vi "Init.vi"(6 "parametrs ref":refnum<vi>, 7 "IP Adress in":string="192.168.0.200", 8 "Stop Event":refnum<user-event>, 9 "control_Pair ref":refnum<vi>, 10 "control_Port_2 ref":refnum<vi>, 11 "control_Port_1 ref":refnum<vi>) -> (0 "error out":errorcluster, 3 "Управление ПЛК":T1)   [LabVIEW 2023, in "pump_Lib.lvlib"]
uses:
  pump_Lib.lvlib
  TypeDef/control_Type.ctl
  TypeDef/pump_Type.ctl
  TypeDef/pair_Type.ctl
  TypeDef/parametrs_Type.ctl
panel:
  # "%"
  # "%"
  # "%"
  # "%"
  # "%"
  # "%"
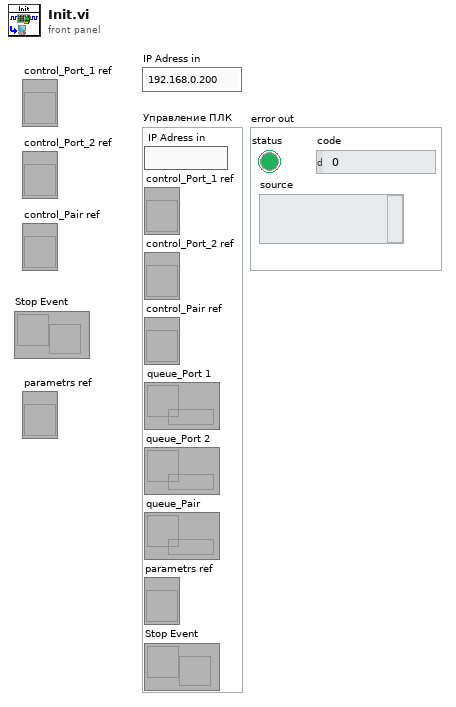
[diagram p1: front panel]
types:
  T1 = typedef "pump_Lib.lvlib/control_Type.ctl" = cluster{"IP Adress in":string, "control_Port_1 ref":refnum<vi>, "control_Port_2 ref":refnum<vi>, "control_Pair ref":refnum<vi>, "queue_Port 1":refnum<queue>, "queue_Port 2":refnum<queue>, "queue_Pair":refnum<queue>, "parametrs ref":refnum<vi>, "Stop Event":refnum<user-event>}
  T2 = typedef "pump_Lib.lvlib/pump_Type.ctl" = cluster{"Давление заданное":dbl, "Давление MAX заданное":dbl, "Давление в насосе":dbl, "Давление в системе":dbl, "Расход заданый":dbl, "Расход текущий":dbl, "Объём заданный":dbl, "Объём текущий":dbl, "Позиция насоса %":dbl, "Ток двигателя":dbl, "controlMsg":string, "Клапан k_sys":bool, "Клапан k_res":bool, "Клапан k_air":bool, "Вверх":bool, "Домой":bool, "Вниз":bool, "Старт расход":bool, "Старт давление":bool, "Сброс объёма":bool, "Сброс давления Рсис":bool, "Сброс давления Рнас":bool, "Bits":cluster{"plc_control":bool, "lag_control":bool, "mstop_control":bool, "st_home":bool, "error":bool, "mstart":bool, "pair":bool, "startQ":bool, "startP":bool, "volume_Stop":bool}}
  T3 = typedef "pump_Lib.lvlib/pair_Type.ctl" = cluster{"Давление заданное":dbl, "Давление в системе":dbl, "Расход заданый":dbl, "Расход текущий":dbl, "Объём заданный":dbl, "Объём текущий":dbl, "Старт давление":bool, "Старт расход":bool, "Сброс объёма":bool, "plc_control":bool, "lag_control":bool, "mstop_control":bool, "Давление":cluster{"АЦП CH 0":dbl, "АЦП CH 1":dbl, "АЦП CH 2":dbl, "АЦП CH 3":dbl, "АЦП CH 4":dbl, "АЦП CH 5":dbl, "АЦП CH 6":dbl, "АЦП CH 7":dbl}, "Modbus":cluster{"Массив чтения":u16[], "Массив записи":u16[]}}
  T4 = enum16{"open", "replace", "create", "open or create", "replace or create", "replace or create with confirmation"}
  T5 = enum16{"big-endian, network order", "native, host order", "little-endian"}
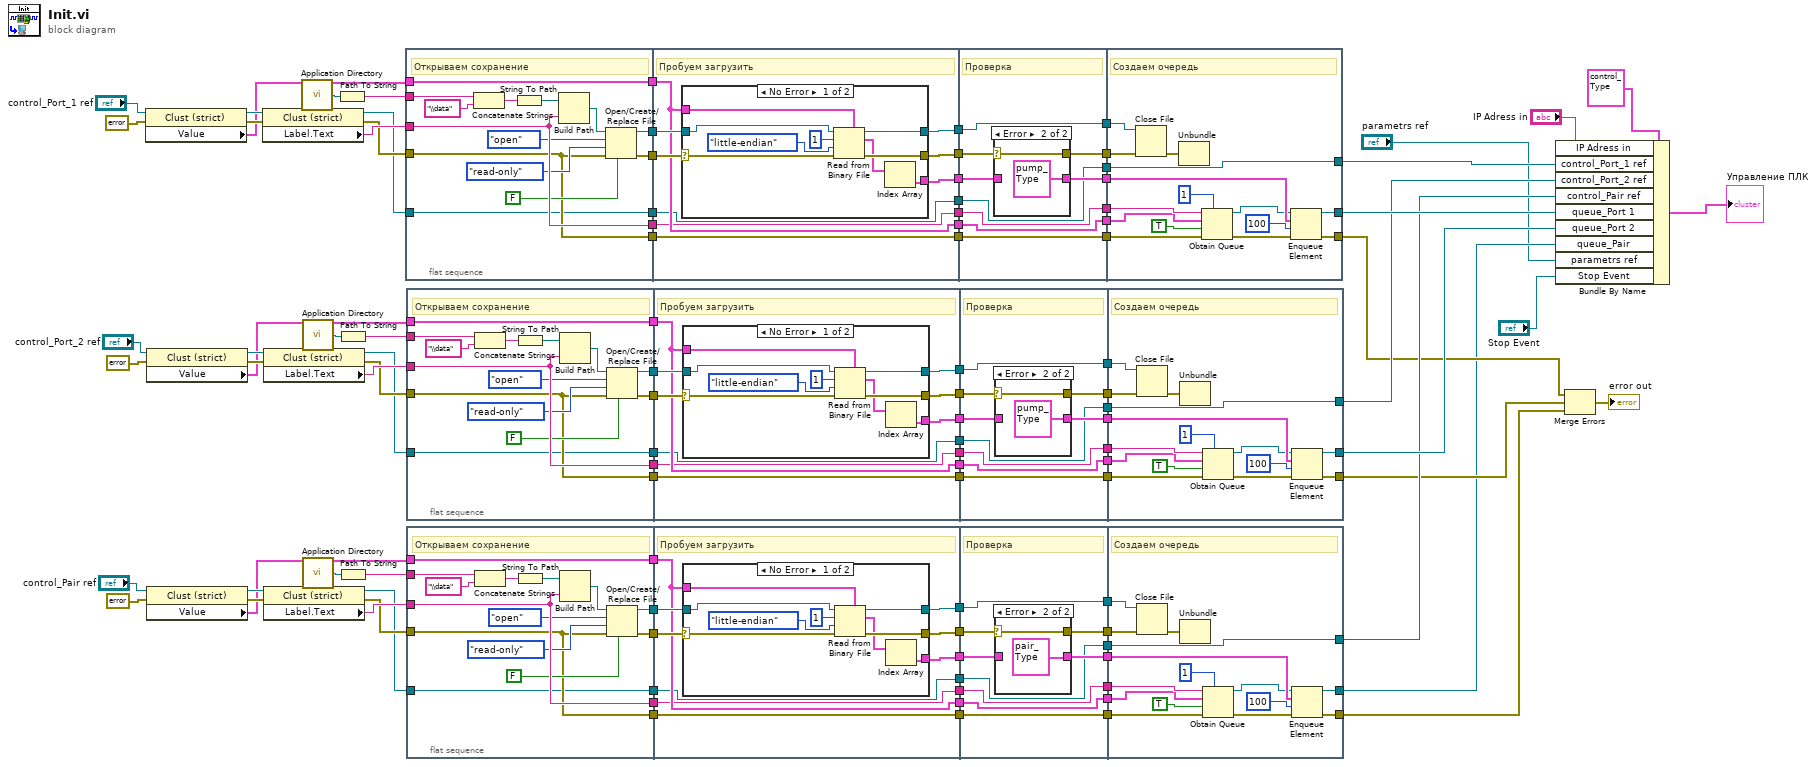
[diagram p0: block diagram]
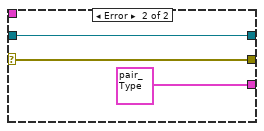
[diagram p2: hidden frame]
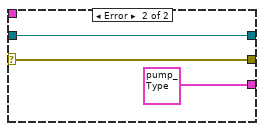
[diagram p4: hidden frame]
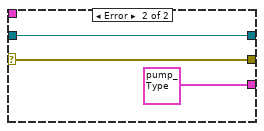
[diagram p6: hidden frame]
diagram:
  n1 = property class="Clust (strict)"(reference="control_Port_1 ref", error in=errorcluster {"status"=FALSE, "code"=0, "source"=""} ("error in (no error)")) -> (reference out=w99:refnum<vi>, error out=w100:errorcluster, "Value"=w77:T2)
  n2 = property class="Clust (strict)"(reference="control_Port_2 ref", error in=errorcluster {"status"=FALSE, "code"=0, "source"=""} ("error in (no error)")) -> (reference out=w47:refnum<vi>, error out=w48:errorcluster, "Value"=w45:T2)
  n3 = property class="Clust (strict)"(reference="control_Pair ref", error in=errorcluster {"status"=FALSE, "code"=0, "source"=""} ("error in (no error)")) -> (reference out=w18:refnum<vi>, error out=w19:errorcluster, "Value"=w16:T3)
  n4 = property class="Clust (strict)"(reference=w99, error in=w100) -> (reference out=w73:refnum<vi>, error out=w74:errorcluster, "Label.Text"=w76:string)
  n5 = property class="Clust (strict)"(reference=w47, error in=w48) -> (reference out=w42:refnum<vi>, error out=w43:errorcluster, "Label.Text"=w44:string)
  n6 = property class="Clust (strict)"(reference=w18, error in=w19) -> (reference out=w13:refnum<vi>, error out=w14:errorcluster, "Label.Text"=w15:string)
  n7 = call <vilib>:"Application Directory.vi"() -> ("Application Directory"=w102:path)
  n8 = call <vilib>:"Application Directory.vi"() -> ("Application Directory"=w50:path)
  n9 = call <vilib>:"Application Directory.vi"() -> ("Application Directory"=w21:path)
  n10 = Path To String(path=w102) -> (string=w78:string)
  n11 = Path To String(path=w50) -> (string=w46:string)
  n12 = Path To String(path=w21) -> (string=w17:string)
  n13 = flat-sequence {
    tunnel: w76 -> [w115]
    tunnel: [w115] -> w98
    tunnel: [w119] -> w97
    tunnel: w77 -> [w119]
    tunnel: w74 -> [w108]
    tunnel: w78 -> [w118]
    tunnel: [w110] -> w96
    tunnel: [w109] -> w95
    tunnel: [w108] -> w94
    tunnel: w73 -> [w106]
    tunnel: [w106] -> w93
    tunnel: w98 -> [w125]
    tunnel: w97 -> [w126]
    tunnel: w96 -> [w128]
    tunnel: w95 -> [w127]
    tunnel: [w126] -> w92
    tunnel: [w125] -> w91
    tunnel: [w124] -> w90
    tunnel: [w123] -> w89
    tunnel: [w122] -> w88
    tunnel: w94 -> [w122]
    tunnel: [w121] -> w87
    tunnel: w93 -> [w121]
    tunnel: [w120] -> w86
    tunnel: w92 -> [w149]
    tunnel: w91 -> [w148]
    tunnel: w90 -> [w146]
    tunnel: w89 -> [w147]
    tunnel: [w149] -> w85
    tunnel: [w148] -> w84
    tunnel: [w145] -> w83
    tunnel: w88 -> [w145]
    tunnel: [w144] -> w82
    tunnel: [w143] -> w81
    tunnel: w87 -> [w143]
    tunnel: [w142] -> w80
    tunnel: [w141] -> w79
    tunnel: w86 -> [w141]
    tunnel: w85 -> [w166]
    tunnel: w84 -> [w167]
    tunnel: w83 -> [w164]
    tunnel: w82 -> [w163]
    tunnel: w81 -> [w158]
    tunnel: [w160] -> w6
    tunnel: [w159] -> w72
    tunnel: [w158] -> w71
    tunnel: w80 -> [w157]
    tunnel: w79 -> [w156]
    frame #0 {
      # "Открываем сохранение"
      n14 = Concatenate Strings(w118, "\\data" ("string")) -> (w117:string)
      n15 = String To Path(string=w117) -> (path=w107:path)
      n16 = Build Path(base path=w107, name or relative path=w115) -> (appended path=w114:path)
      n17 = Open/Create/Replace File(file path (use dialog)=w114, error in=w108, operation (0:open)=T4."open", access (0:read/write)=enum16{"read/write", "read-only", "write-only"}."read-only", disable buffering (F)=FALSE) -> (refnum out=w109:refnum<file>, error out=w110:errorcluster)  [unwired: 1 in, 1 out]
    }
    frame #1 {
      # "Пробуем загрузить"
      n18 = case shown="No Error" w128 {
        selector: w128 -> [w136 w140]
        tunnel: w127 -> [w137 w139]
        tunnel: w126 -> [w135 _]
        tunnel: [w130 T2 {"Давление заданное"=0.3, "Давление MAX заданное"=100.0, "Давление в насосе"=0.0, "Давление в системе"=99.99, "Расход заданый"=0.0, "Расход текущий"=0.0, "Объём заданный"=0.0, "Объём текущий"=0.0, "Позиция насоса %"=0.0, "Ток двигателя"=0.0, "controlMsg"="", "Клапан k_sys"=FALSE, "Клапан k_res"=FALSE, "Клапан k_air"=FALSE, "Вверх"=FALSE, "Домой"=FALSE, "Вниз"=FALSE, "Старт расход"=FALSE, "Старт давление"=FALSE, "Сброс объёма"=FALSE, "Сброс давления Рсис"=FALSE, "Сброс давления Рнас"=FALSE, "Bits"={"plc_control"=FALSE, "lag_control"=FALSE, "mstop_control"=FALSE, "st_home"=FALSE, "error"=FALSE, "mstart"=FALSE, "pair"=FALSE, "startQ"=FALSE, "startP"=FALSE, "volume_Stop"=FALSE}} ("Насос")] -> w124
        tunnel: [w132 w140] -> w123
        tunnel: [w129 w139] -> w120
        frame No Error {
          n19 = Read from Binary File(5:w135, 8:w136, 9:T5."little-endian" ("byte order (0:big-endian, network order)"), 10:1 ("count (1)"), 11:w137) -> (0:w132:errorcluster, 2:w131:T2[], 3:w129:refnum<file>)  [unwired: 1 in, 1 out]
          n20 = Index Array(array=w131) -> (element=w130:T2)  [unwired: 1 in]
        }
        frame Error {
        }
      }
    }
    frame #2 {
      # "Проверка"
      n21 = case shown="Error" w147 {
        selector: w147 -> [w150 w153]
        tunnel: w146 -> [w151 _]
        tunnel: [w151 T2 {"Давление заданное"=0.3, "Давление MAX заданное"=100.0, "Давление в насосе"=0.0, "Давление в системе"=99.99, "Расход заданый"=0.0, "Расход текущий"=0.0, "Объём заданный"=0.0, "Объём текущий"=0.0, "Позиция насоса %"=0.0, "Ток двигателя"=0.0, "controlMsg"="", "Клапан k_sys"=FALSE, "Клапан k_res"=FALSE, "Клапан k_air"=FALSE, "Вверх"=FALSE, "Домой"=FALSE, "Вниз"=FALSE, "Старт расход"=FALSE, "Старт давление"=FALSE, "Сброс объёма"=FALSE, "Сброс давления Рсис"=FALSE, "Сброс давления Рнас"=FALSE, "Bits"={"plc_control"=FALSE, "lag_control"=FALSE, "mstop_control"=FALSE, "st_home"=FALSE, "error"=FALSE, "mstart"=FALSE, "pair"=FALSE, "startQ"=FALSE, "startP"=FALSE, "volume_Stop"=FALSE}} ("Насос")] -> w144
        tunnel: [w150 w153] -> w142
        frame No Error {
        }
        frame Error {
        }
      }
    }
    frame #3 {
      # "Создаем очередь"
      n22 = Close File(refnum=w156, error in=w157) -> (error out=w155:errorcluster)  [unwired: 1 out]
      n23 = Unbundle(w155) -> ()  [unwired: 3 out]
      n24 = Obtain Queue(max queue size (-1, unlimited)=1, name (unnamed)=w167, element data type=w166, create if not found? (T)=TRUE, error in (no error)=w164) -> (queue out=w162:refnum<queue>, error out=w161:errorcluster)  [unwired: 1 out]
      n25 = Enqueue Element(queue=w162, element=w163, timeout in ms (-1)=100, error in (no error)=w161) -> (queue out=w159:refnum<queue>, error out=w160:errorcluster)  [unwired: 1 out]
    }
  }
  n26 = flat-sequence {
    tunnel: w44 -> [w178]
    tunnel: [w178] -> w70
    tunnel: [w182] -> w69
    tunnel: w45 -> [w182]
    tunnel: w43 -> [w171]
    tunnel: w46 -> [w181]
    tunnel: [w173] -> w68
    tunnel: [w172] -> w67
    tunnel: [w171] -> w66
    tunnel: w42 -> [w169]
    tunnel: [w169] -> w65
    tunnel: w70 -> [w188]
    tunnel: w69 -> [w189]
    tunnel: w68 -> [w191]
    tunnel: w67 -> [w190]
    tunnel: [w189] -> w64
    tunnel: [w188] -> w63
    tunnel: [w187] -> w62
    tunnel: [w186] -> w61
    tunnel: [w185] -> w60
    tunnel: w66 -> [w185]
    tunnel: [w184] -> w59
    tunnel: w65 -> [w184]
    tunnel: [w183] -> w58
    tunnel: w64 -> [w212]
    tunnel: w63 -> [w211]
    tunnel: w62 -> [w209]
    tunnel: w61 -> [w210]
    tunnel: [w212] -> w57
    tunnel: [w211] -> w56
    tunnel: [w208] -> w55
    tunnel: w60 -> [w208]
    tunnel: [w207] -> w54
    tunnel: [w206] -> w53
    tunnel: w59 -> [w206]
    tunnel: [w205] -> w52
    tunnel: [w204] -> w51
    tunnel: w58 -> [w204]
    tunnel: w57 -> [w229]
    tunnel: w56 -> [w230]
    tunnel: w55 -> [w227]
    tunnel: w54 -> [w226]
    tunnel: w53 -> [w221]
    tunnel: [w223] -> w5
    tunnel: [w222] -> w9
    tunnel: [w221] -> w10
    tunnel: w52 -> [w220]
    tunnel: w51 -> [w219]
    frame #0 {
      # "Открываем сохранение"
      n27 = Concatenate Strings(w181, "\\data" ("string")) -> (w180:string)
      n28 = String To Path(string=w180) -> (path=w170:path)
      n29 = Build Path(base path=w170, name or relative path=w178) -> (appended path=w177:path)
      n30 = Open/Create/Replace File(file path (use dialog)=w177, error in=w171, operation (0:open)=T4."open", access (0:read/write)=enum16{"read/write", "read-only", "write-only"}."read-only", disable buffering (F)=FALSE) -> (refnum out=w172:refnum<file>, error out=w173:errorcluster)  [unwired: 1 in, 1 out]
    }
    frame #1 {
      # "Пробуем загрузить"
      n31 = case shown="No Error" w191 {
        selector: w191 -> [w199 w203]
        tunnel: w190 -> [w200 w202]
        tunnel: w189 -> [w198 _]
        tunnel: [w193 T2 {"Давление заданное"=0.3, "Давление MAX заданное"=100.0, "Давление в насосе"=0.0, "Давление в системе"=99.99, "Расход заданый"=0.0, "Расход текущий"=0.0, "Объём заданный"=0.0, "Объём текущий"=0.0, "Позиция насоса %"=0.0, "Ток двигателя"=0.0, "controlMsg"="", "Клапан k_sys"=FALSE, "Клапан k_res"=FALSE, "Клапан k_air"=FALSE, "Вверх"=FALSE, "Домой"=FALSE, "Вниз"=FALSE, "Старт расход"=FALSE, "Старт давление"=FALSE, "Сброс объёма"=FALSE, "Сброс давления Рсис"=FALSE, "Сброс давления Рнас"=FALSE, "Bits"={"plc_control"=FALSE, "lag_control"=FALSE, "mstop_control"=FALSE, "st_home"=FALSE, "error"=FALSE, "mstart"=FALSE, "pair"=FALSE, "startQ"=FALSE, "startP"=FALSE, "volume_Stop"=FALSE}} ("Насос")] -> w187
        tunnel: [w195 w203] -> w186
        tunnel: [w192 w202] -> w183
        frame No Error {
          n32 = Read from Binary File(5:w198, 8:w199, 9:T5."little-endian" ("byte order (0:big-endian, network order)"), 10:1 ("count (1)"), 11:w200) -> (0:w195:errorcluster, 2:w194:T2[], 3:w192:refnum<file>)  [unwired: 1 in, 1 out]
          n33 = Index Array(array=w194) -> (element=w193:T2)  [unwired: 1 in]
        }
        frame Error {
        }
      }
    }
    frame #2 {
      # "Проверка"
      n34 = case shown="Error" w210 {
        selector: w210 -> [w213 w216]
        tunnel: w209 -> [w214 _]
        tunnel: [w214 T2 {"Давление заданное"=0.3, "Давление MAX заданное"=100.0, "Давление в насосе"=0.0, "Давление в системе"=99.99, "Расход заданый"=0.0, "Расход текущий"=0.0, "Объём заданный"=0.0, "Объём текущий"=0.0, "Позиция насоса %"=0.0, "Ток двигателя"=0.0, "controlMsg"="", "Клапан k_sys"=FALSE, "Клапан k_res"=FALSE, "Клапан k_air"=FALSE, "Вверх"=FALSE, "Домой"=FALSE, "Вниз"=FALSE, "Старт расход"=FALSE, "Старт давление"=FALSE, "Сброс объёма"=FALSE, "Сброс давления Рсис"=FALSE, "Сброс давления Рнас"=FALSE, "Bits"={"plc_control"=FALSE, "lag_control"=FALSE, "mstop_control"=FALSE, "st_home"=FALSE, "error"=FALSE, "mstart"=FALSE, "pair"=FALSE, "startQ"=FALSE, "startP"=FALSE, "volume_Stop"=FALSE}} ("Насос")] -> w207
        tunnel: [w213 w216] -> w205
        frame No Error {
        }
        frame Error {
        }
      }
    }
    frame #3 {
      # "Создаем очередь"
      n35 = Close File(refnum=w219, error in=w220) -> (error out=w218:errorcluster)  [unwired: 1 out]
      n36 = Unbundle(w218) -> ()  [unwired: 3 out]
      n37 = Obtain Queue(max queue size (-1, unlimited)=1, name (unnamed)=w230, element data type=w229, create if not found? (T)=TRUE, error in (no error)=w227) -> (queue out=w225:refnum<queue>, error out=w224:errorcluster)  [unwired: 1 out]
      n38 = Enqueue Element(queue=w225, element=w226, timeout in ms (-1)=100, error in (no error)=w224) -> (queue out=w222:refnum<queue>, error out=w223:errorcluster)  [unwired: 1 out]
    }
  }
  n39 = flat-sequence {
    tunnel: w15 -> [w241]
    tunnel: [w241] -> w41
    tunnel: [w245] -> w40
    tunnel: w16 -> [w245]
    tunnel: w14 -> [w234]
    tunnel: w17 -> [w244]
    tunnel: [w236] -> w39
    tunnel: [w235] -> w38
    tunnel: [w234] -> w37
    tunnel: w13 -> [w232]
    tunnel: [w232] -> w36
    tunnel: w41 -> [w251]
    tunnel: w40 -> [w252]
    tunnel: w39 -> [w254]
    tunnel: w38 -> [w253]
    tunnel: [w252] -> w35
    tunnel: [w251] -> w34
    tunnel: [w250] -> w33
    tunnel: [w249] -> w32
    tunnel: [w248] -> w31
    tunnel: w37 -> [w248]
    tunnel: [w247] -> w30
    tunnel: w36 -> [w247]
    tunnel: [w246] -> w29
    tunnel: w35 -> [w275]
    tunnel: w34 -> [w274]
    tunnel: w33 -> [w272]
    tunnel: w32 -> [w273]
    tunnel: [w275] -> w28
    tunnel: [w274] -> w27
    tunnel: [w271] -> w26
    tunnel: w31 -> [w271]
    tunnel: [w270] -> w25
    tunnel: [w269] -> w24
    tunnel: w30 -> [w269]
    tunnel: [w268] -> w23
    tunnel: [w267] -> w22
    tunnel: w29 -> [w267]
    tunnel: w28 -> [w292]
    tunnel: w27 -> [w293]
    tunnel: w26 -> [w290]
    tunnel: w25 -> [w289]
    tunnel: w24 -> [w284]
    tunnel: [w286] -> w4
    tunnel: [w285] -> w3
    tunnel: [w284] -> w8
    tunnel: w23 -> [w283]
    tunnel: w22 -> [w282]
    frame #0 {
      # "Открываем сохранение"
      n40 = Concatenate Strings(w244, "\\data" ("string")) -> (w243:string)
      n41 = String To Path(string=w243) -> (path=w233:path)
      n42 = Build Path(base path=w233, name or relative path=w241) -> (appended path=w240:path)
      n43 = Open/Create/Replace File(file path (use dialog)=w240, error in=w234, operation (0:open)=T4."open", access (0:read/write)=enum16{"read/write", "read-only", "write-only"}."read-only", disable buffering (F)=FALSE) -> (refnum out=w235:refnum<file>, error out=w236:errorcluster)  [unwired: 1 in, 1 out]
    }
    frame #1 {
      # "Пробуем загрузить"
      n44 = case shown="No Error" w254 {
        selector: w254 -> [w262 w266]
        tunnel: w253 -> [w263 w265]
        tunnel: w252 -> [w261 _]
        tunnel: [w256 T3 {"Давление заданное"=0.3, "Давление в системе"=99.99, "Расход заданый"=0.0, "Расход текущий"=0.0, "Объём заданный"=0.0, "Объём текущий"=0.0, "Старт давление"=FALSE, "Старт расход"=FALSE, "Сброс объёма"=FALSE, "plc_control"=FALSE, "lag_control"=FALSE, "mstop_control"=FALSE, "Давление"={"АЦП CH 0"=0.0, "АЦП CH 1"=0.0, "АЦП CH 2"=0.0, "АЦП CH 3"=0.0, "АЦП CH 4"=0.0, "АЦП CH 5"=0.0, "АЦП CH 6"=0.0, "АЦП CH 7"=0.0}, "Modbus"={"Массив чтения"=[], "Массив записи"=[]}} ("Насосная система")] -> w250
        tunnel: [w258 w266] -> w249
        tunnel: [w255 w265] -> w246
        frame No Error {
          n45 = Read from Binary File(5:w261, 8:w262, 9:T5."little-endian" ("byte order (0:big-endian, network order)"), 10:1 ("count (1)"), 11:w263) -> (0:w258:errorcluster, 2:w257:T3[], 3:w255:refnum<file>)  [unwired: 1 in, 1 out]
          n46 = Index Array(array=w257) -> (element=w256:T3)  [unwired: 1 in]
        }
        frame Error {
        }
      }
    }
    frame #2 {
      # "Проверка"
      n47 = case shown="Error" w273 {
        selector: w273 -> [w276 w279]
        tunnel: w272 -> [w277 _]
        tunnel: [w277 T3 {"Давление заданное"=0.3, "Давление в системе"=99.99, "Расход заданый"=0.0, "Расход текущий"=0.0, "Объём заданный"=0.0, "Объём текущий"=0.0, "Старт давление"=FALSE, "Старт расход"=FALSE, "Сброс объёма"=FALSE, "plc_control"=FALSE, "lag_control"=FALSE, "mstop_control"=FALSE, "Давление"={"АЦП CH 0"=0.0, "АЦП CH 1"=0.0, "АЦП CH 2"=0.0, "АЦП CH 3"=0.0, "АЦП CH 4"=0.0, "АЦП CH 5"=0.0, "АЦП CH 6"=0.0, "АЦП CH 7"=0.0}, "Modbus"={"Массив чтения"=[], "Массив записи"=[]}} ("Насосная система")] -> w270
        tunnel: [w276 w279] -> w268
        frame No Error {
        }
        frame Error {
        }
      }
    }
    frame #3 {
      # "Создаем очередь"
      n48 = Close File(refnum=w282, error in=w283) -> (error out=w281:errorcluster)  [unwired: 1 out]
      n49 = Unbundle(w281) -> ()  [unwired: 3 out]
      n50 = Obtain Queue(max queue size (-1, unlimited)=1, name (unnamed)=w293, element data type=w292, create if not found? (T)=TRUE, error in (no error)=w290) -> (queue out=w288:refnum<queue>, error out=w287:errorcluster)  [unwired: 1 out]
      n51 = Enqueue Element(queue=w288, element=w289, timeout in ms (-1)=100, error in (no error)=w287) -> (queue out=w285:refnum<queue>, error out=w286:errorcluster)  [unwired: 1 out]
    }
  }
  n52 = Bundle By Name(cluster=T1 {"IP Adress in"="", "control_Port_1 ref"=refnum, "control_Port_2 ref"=refnum, "control_Pair ref"=refnum, "queue_Port 1"=refnum, "queue_Port 2"=refnum, "queue_Pair"=refnum, "parametrs ref"=refnum, "Stop Event"=refnum} ("Управление ПЛК"), "IP Adress in"="IP Adress in", "control_Port_1 ref"=w71, "control_Port_2 ref"=w10, "control_Pair ref"=w8, "queue_Port 1"=w72, "queue_Port 2"=w9, "queue_Pair"=w3, "parametrs ref"="parametrs ref", "Stop Event"="Stop Event") -> (→"Управление ПЛК":T1)
  n53 = Merge Errors(w6, w5, w4) -> (→"error out":errorcluster)
